vi "make default test sequence.vi"(8 "error in":errorcluster, 11 "file path":path) -> (0 "error out":errorcluster, 3 "new file path":path)   [LabVIEW 2021]
uses:
  controls/developer_test sequence.ctl
  controls/test type selection.ctl
  controls/comparison selection.ctl
  controls/test step description.ctl
  <vilib>/Utility/file.llb/Write Delimited Spreadsheet (string).vi
panel:
  in  "Comparison":T1=enum."greater or equal to?" caption="Enum"
  in  "test type":T2 caption="Enum"
  in  "developer_test sequence":T3=enum."Report" caption="Enum"
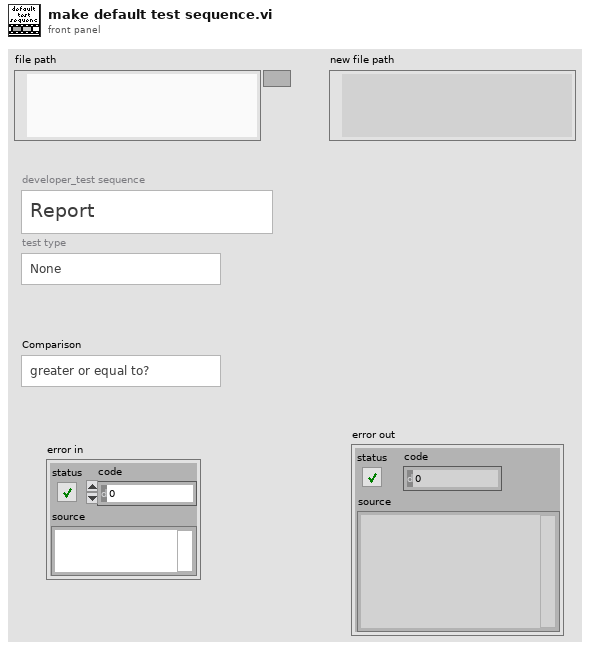
[diagram p1: front panel]
types:
  T1 = typedef "comparison selection.ctl" = enum16{"None", "in-range?", "less than?", "greater than?", "equal to?", "not equal to?", "less or equal to?", "greater or equal to?"}
  T2 = typedef "test type selection.ctl" = enum16{"None", "Voltage", "Voltage?", "Current", "Current?", "Output", "Program"}
  T3 = typedef "developer_test sequence.ctl" = enum16{"Update Display", "User Login", "Initialise", "Init Devices", "Idle State", "test steup", "Abort", "Start Display Board Auto Testing", "Scan Barcode", "Checking TEMP at Thermistor 1", "Checking TEMP at Thermistor 2", "Checking TEMP at Thermistor 3", "Checking TEMP at Thermistor 4 (Ambient)", "Voltage Health Check", "INSULATION Resistance test (Baseplate to Negative)", "INSULATION Resistance test (Baseplate to Positive)", "WELD Resistance Test", "Stop Display Board Auto Testing", "All Pass", "Fail", "Report", "Error", "Confirm Quit", "Exit"}
  T4 = typedef "test step description.ctl" = cluster{"test type":T2, "developer_test sequence":T3, "Lower limit":dbl, "Upper limit":dbl, "Comparison":T1}
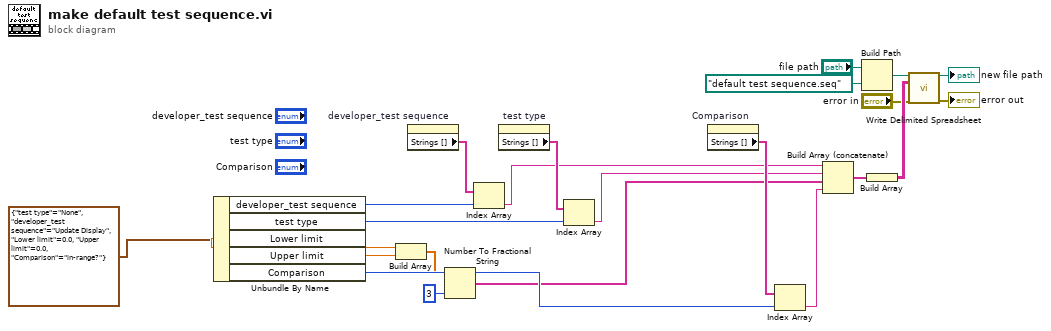
[diagram p0: block diagram]
diagram:
  n1 = Unbundle By Name(T4 {"test type"=enum."None", "developer_test sequence"=enum."Update Display", "Lower limit"=0.0, "Upper limit"=0.0, "Comparison"=enum."in-range?"} ("test tsep description")) -> ("developer_test sequence"=w20:T3, "test type"=w19:T2, "Lower limit"=w17:dbl, "Upper limit"=w16:dbl, "Comparison"=w18:T1)
  n2 = Build Array(w17, w16) -> (w15:dbl[])
  n3 = property on="developer_test sequence" class="Enum (strict)"() -> ("Strings []"=w23:string[])  [unwired: 2 in, 2 out]
  n4 = Number To Fractional String(number=w15, precision (6)=i16 3) -> (F-format string=w3:string[])  [unwired: 2 in]
  n5 = Index Array(array=w23, index=w20) -> (element=w14:string)
  n6 = property on="test type" class="Enum (strict)"() -> ("Strings []"=w22:string[])  [unwired: 2 in, 2 out]
  n7 = Index Array(array=w22, index=w19) -> (element=w13:string)
  n8 = property on="Comparison" class="Enum (strict)"() -> ("Strings []"=w21:string[])  [unwired: 2 in, 2 out]
  n9 = Index Array(array=w21, index=w18) -> (element=w2:string)
  n10 = Build Array (concatenate)(w14, w13, w3, w2) -> (w7:string[])
  n11 = Build Path(base path="file path", name or relative path=path "default test sequence.seq") -> (appended path=w10:path)
  n12 = Build Array(w7) -> (w6:string[][])
  n13 = call-poly <vilib>:"Write Delimited Spreadsheet.vi"("file path (dialog if empty)"=w10, "2D data"=w6, "error in (no error)"="error in") -> ("new file path (Not A Path if cancelled)"=→"new file path":path, "error out"=→"error out":errorcluster)  [unwired: 11 in]
